vi "pumpdialog.vi"() -> (1 "amplitude (volts)":dbl format="%.2f", 2 "waveform":sgl[](array[numeric]) format="%.2f", 3 "new file path":path)   [LabVIEW 2010]
uses:
  <vilib>/Utility/file.llb/Write To Spreadsheet File (DBL).vi
panel:
  in  "conversion (volts/(m3/s)":sgl=1.0 format="%.2f"
  in  "stop":bool
  in  "Get Wave":bool
  out "graph":dbl[](graph)
  in  "flow (m3/s)":sgl=1.0 min=0 max=8.4 format="%.2f"
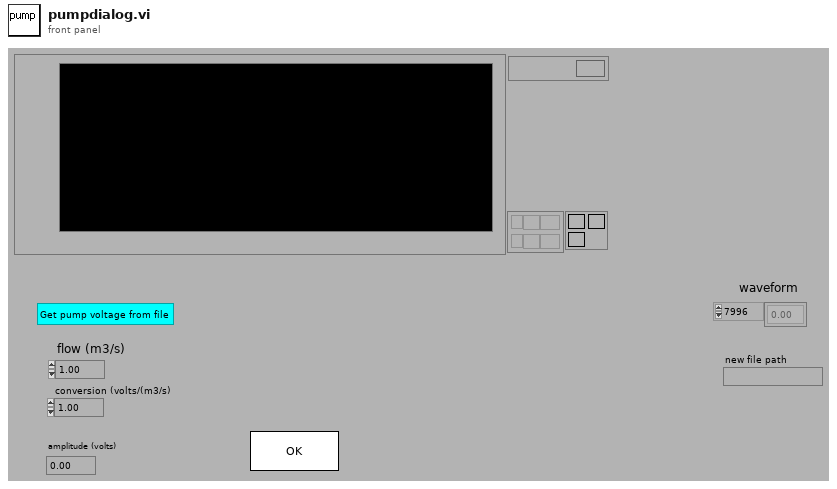
[diagram p1: front panel]
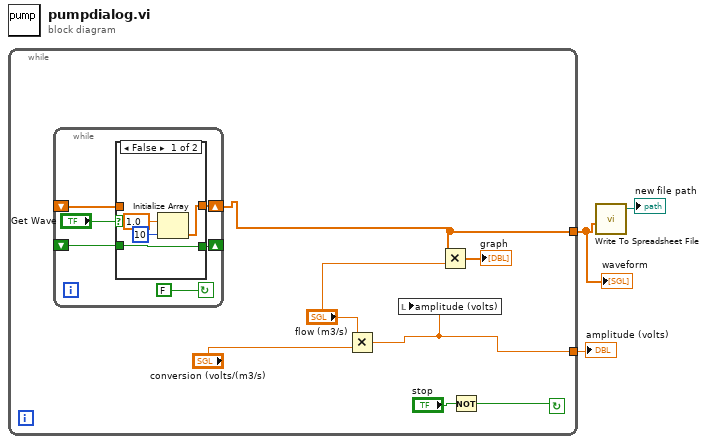
[diagram p0: block diagram]
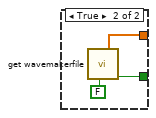
[diagram p2: hidden frame]
diagram:
  n1 = while {
    tunnel: [w5] -> w1
    tunnel: [w6] -> w2
    stop <- w10 continue-if-true
    n2 = while {
      shift-left: _ -> [w12]
      shift-right: [w13] -> _
      shift-left: _ -> [w15]
      shift-right: [w14] -> w5
      stop <- FALSE continue-if-true
      n3 = case shown="False" "Get Wave" {
        tunnel: [w19 w22] -> w14
        tunnel: w15 -> [_ _]
        tunnel: [w20 w21] -> w13
        tunnel: w12 -> [w20 _]
        frame False {
          n4 = Initialize Array(1.0 ("Element Data"), 10 ("Dimension Size")) -> (w19:dbl[])
        }
        frame True {
          n5 = call "get wavemakerfile.vi"("warning"=FALSE) -> ("discontinuities"=w21:bool, "waveform"=w22:sgl[])  [unwired: 8 in, 1 out]
        }
      }
    }
    n6 = Multiply(x="flow (m3/s)", y="conversion (volts/(m3/s)") -> (x*y=w6:sgl)
    n7 = local write "amplitude (volts)"(w6) -> ()
    n8 = Multiply(x=w5, y="flow (m3/s)") -> (x*y=→"graph":dbl[])
    n9 = Not(x="stop") -> (.not. x?=w10:bool)
  }
  "amplitude (volts)" <- w2
  "waveform" <- w1
  n10 = call-poly <vilib>:"Write To Spreadsheet File.vi"("1D data"=w1) -> ("new file path (Not A Path if cancelled)"=→"new file path":path)  [unwired: 7 in]
